vi "Configure Output.vi"(8 "error in (no error)":errorcluster, 11 "FGen PXI Base CFG in":refnum<class "FGen PXI Base CFG.lvclass">) -> (0 "error out":errorcluster, 3 "FGen PXI Base CFG out":refnum<class "FGen PXI Base CFG.lvclass">)   [LabVIEW 2023, in "FGen PXI Base CFG.lvlib" / "FGen PXI Base CFG.lvclass"]
uses:
  FGen PXI Base CFG.lvclass
  7d5647a1-ee57-477e-af02-dfb71140fe97.vi
  <vilib>/ErrorRing/Error Ring.xnode
  <vilib>/Utility/error.llb/Error Cluster From Error Code.vi
  Configuration/Configuration JSON/Configuration JSON Base/CFG JSON.lvclass
  D:/git/HAL/HAL GOOP4/FGen/FGen Base CFG/FGen Base CFG.lvclass
  D:/git/HAL/HAL GOOP4/Configuration JSON Base/CFG JSON.lvclass
  D:/git/HAL/HAL GOOP4/Interfaces/IConfigure/IConfigure.lvclass
  D:/git/HAL/HAL GOOP4/FGen/FGen PXI/FGen PXI Base CFG/FGen PXI Base CFG.lvclass
panel:
  out "Advanced:Idle Behavior":i32(ring)=400 items=["Hold Last Value"=400, "Jump To Value"=401]
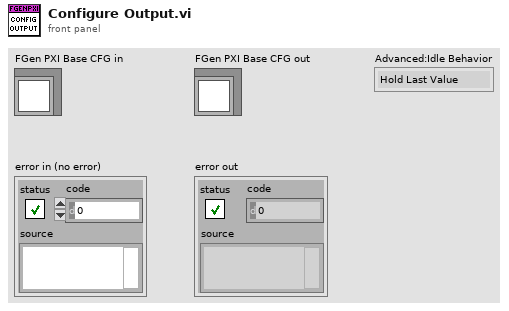
[diagram p1: front panel]
types:
  T1 = cluster{"Idle Behavior":string, "Idle Value":i32, "Digital Gain":dbl}
  T2 = typedef "LVStringsAndValuesArrayTypeDef_I32.ctl" = cluster{"String":string, "Value":i32}[]
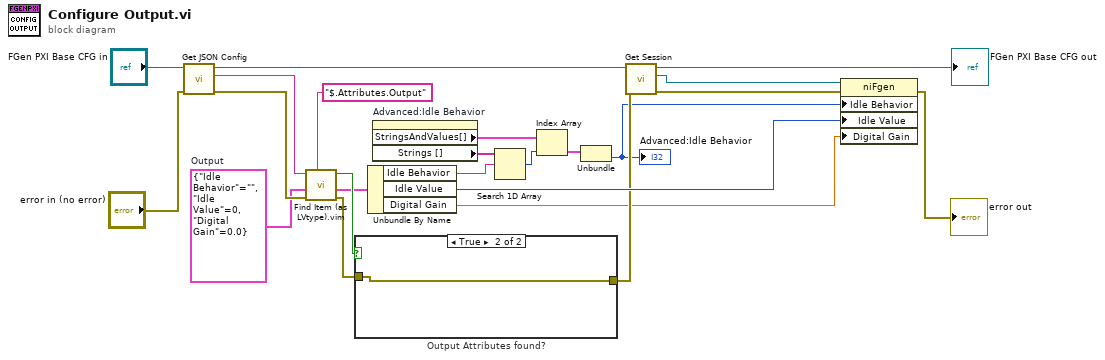
[diagram p0: block diagram]
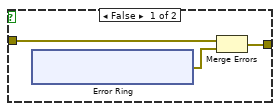
[diagram p2: hidden frame]
diagram:
  w15 = T1 {"Idle Behavior"="", "Idle Value"=0, "Digital Gain"=0.0}  # Output
  n1 = call "Get JSON Config.vi"("error in (no error)"="error in (no error)", "CFG Base in"="FGen PXI Base CFG in") -> ("error out"=w16:errorcluster, "<JSON>Config>"=w17:string, "CFG Base out"=w19:refnum<class "FGen PXI Base CFG.lvclass">)  [unwired: 7 in]
  n2 = call "Find Item (as LVtype).vim"("$Path or Item Name"="$.Attributes.Output", "error in (no error)"=w16, "Data Type and Default Value"=w15, "JSON"=w17) -> ("error out"=w13:errorcluster, "Data"=w12:T1, "Found"=w14:bool)  [unwired: 4 in, 1 out]
  n3 = case "Output Attributes found?" shown="True" w14 {
    tunnel: w13 -> [w26 w32]
    tunnel: [w24 w32] -> w6
    frame False {
      n4 = xnode "Error Ring"() -> ("error out"=w25:errorcluster)
      n5 = Merge Errors(w26, w25) -> (w24:errorcluster)
    }
    frame True {
    }
  }
  n6 = Unbundle By Name(w12) -> ("Idle Behavior"=w11:string, "Idle Value"=w7:i32, "Digital Gain"=w1:dbl)
  n7 = property on="Advanced:Idle Behavior" class="Ring (strict)"() -> ("StringsAndValues[]"=w10:T2, "Strings []"=w21:string[])  [unwired: 2 in, 2 out]
  n8 = Search 1D Array(1D array=w21, element=w11) -> (index of element=w5:i32)  [unwired: 1 in]
  n9 = Index Array(array=w10, index=w5) -> (element=w9:cluster{"String":string, "Value":i32})
  n10 = Unbundle(w9) -> ("Value"=w3:i32)  [unwired: 1 out]
  "Advanced:Idle Behavior" <- w3
  n11 = call "Get Session.vi"("error in (no error)"=w6, "FGen PXI Base CFG in"=w19) -> ("error out"=w8:errorcluster, "Session"=w22:refnum<k15>, "FGen PXI Base CFG out"=→"FGen PXI Base CFG out":refnum<class "FGen PXI Base CFG.lvclass">)  [unwired: 7 in]
  n12 = property class="niFgen"(reference=w22, error in=w8, "Idle Behavior"=w3, "Idle Value"=w7, "Digital Gain"=w1) -> (error out=→"error out":errorcluster)  [unwired: 1 out]
